vi "Init.vi"(8 "error in (no error)":errorcluster, 11 "reference in":refnum<class "Test_Flux_Capacitor.lvclass">) -> (0 "error out":errorcluster, 3 "reference out":refnum<class "Test_Flux_Capacitor.lvclass">)   [LabVIEW 2022 SP3, in "Test_Flux_Capacitor.lvlib" / "Test_Flux_Capacitor.lvclass"]
uses:
  Test_Flux_Capacitor.lvclass
  Components/Test_Base.lvlibp/Test_Base.lvclass
  Components/ViPER.lvlibp/ViPER.lvclass
  C:/Projects/Medulla/ViPER/Examples/Flux_Capacitor_Tester/Components/ViPER.lvlibp/ViPER.lvclass
  Components/Flux_Capacitor.lvlibp/Flux_Capacitor.lvclass
  Components/SwitchBase.lvlibp/SwitchBase.lvclass
  Components/PSU_Base.lvlibp/PSU_Base.lvclass
  Components/LCR_BK891.lvlibp/LCR_BK891.lvclass
  Components/DMM_Keysight_34980A.lvlibp/DMM_Keysight_34980A.lvclass
  Components/JTAG_Base.lvlibp/JTAG_Base.lvclass
  Components/Frequency_Counter_Base.lvlibp/Frequency_Counter_Base.lvclass
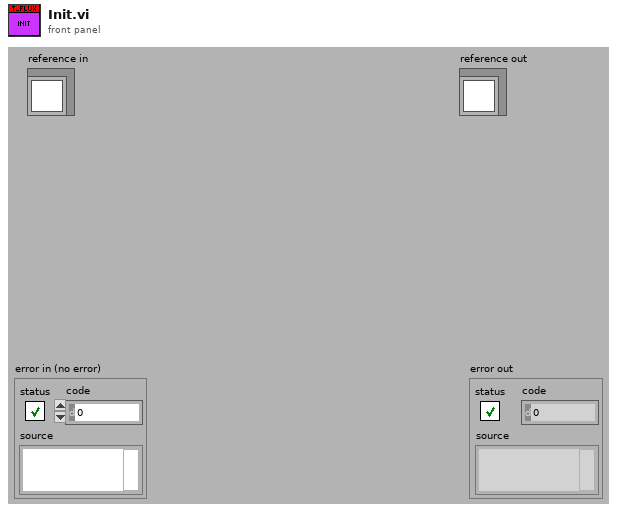
[diagram p1: front panel]
types:
  T1 = typedef "Test_Flux_Capacitor.lvlib/Test_Flux_Capacitor.lvclass/ObjectAttributes.ctl" = cluster{"Config":T2, "DMM":refnum<class "DMM_Keysight_34980A.lvclass">, "LCR":refnum<class "LCR_BK891.lvclass">, "PSU":refnum<class "PSU_Base.lvclass">, "Switch_Manager":refnum<class "SwitchBase.lvclass">, "FRAM":string, "Flux_Capacitor":refnum<class "Flux_Capacitor.lvclass">, "Frequency_Counter":refnum<class "Frequency_Counter_Base.lvclass">, "JTAG":refnum<class "JTAG_Base.lvclass">}
  T2 = typedef "Test_Flux_Capacitor.lvlib/Test_Flux_Capacitor.lvclass/Config.ctl" = cluster{"default":string}
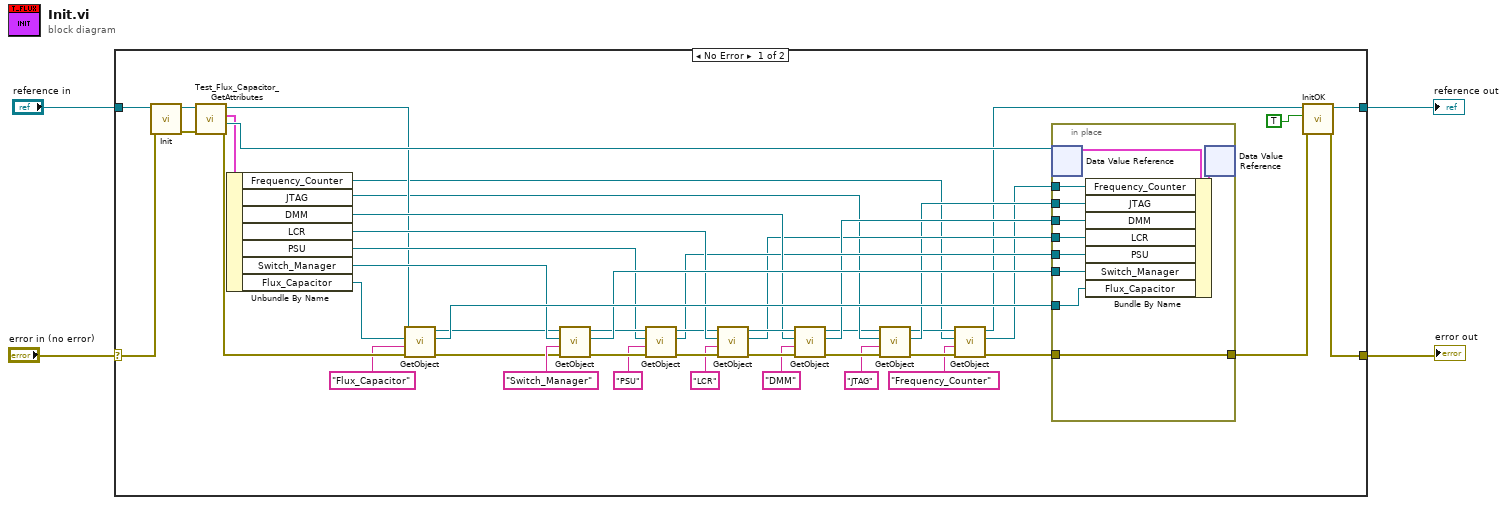
[diagram p0: block diagram]
diagram:
  n1 = case shown="No Error" "error in (no error)" {
    selector: "error in (no error)" -> [w50 w63]
    tunnel: [w43 w63] -> w3
    tunnel: [w46 w62] -> w1
    tunnel: "reference in" -> [w51 w62]
    frame No Error {
      n2 = call-parent "Init.vi"("error in (no error)"=w50, "reference in"=w51) -> ("error out"=w48:errorcluster, "reference out"=w49:refnum<class "Test_Flux_Capacitor.lvclass">)  [unwired: 8 in]
      n3 = call "Test_Flux_Capacitor_GetAttributes.vi"("error in (no error)"=w48, "reference in"=w49) -> ("error out"=w42:errorcluster, "DataRef"=w47:refnum<data-value>, "Data"=w41:T1, "reference out"=w19:refnum<class "Test_Flux_Capacitor.lvclass">)  [unwired: 6 in]
      n4 = Unbundle By Name(w41) -> ("Frequency_Counter"=w8:refnum<class "Frequency_Counter_Base.lvclass">, "JTAG"=w15:refnum<class "JTAG_Base.lvclass">, "DMM"=w24:refnum<class "DMM_Keysight_34980A.lvclass">, "LCR"=w29:refnum<class "LCR_BK891.lvclass">, "PSU"=w32:refnum<class "PSU_Base.lvclass">, "Switch_Manager"=w37:refnum<class "SwitchBase.lvclass">, "Flux_Capacitor"=w40:refnum<class "Flux_Capacitor.lvclass">)
      n5 = call "GetObject.vi"("error in (no error)"=w42, "Object Name"="Flux_Capacitor", "Class type"=w40, "reference in"=w19) -> ("error out"=w18:errorcluster, "Object out"=w38:refnum<class "Flux_Capacitor.lvclass">, "reference out"=w17:refnum<class "Test_Flux_Capacitor.lvclass">)  [unwired: 5 in]
      n6 = call "GetObject.vi"("error in (no error)"=w18, "Object Name"="Switch_Manager", "Class type"=w37, "reference in"=w17) -> ("error out"=w34:errorcluster, "Object out"=w35:refnum<class "SwitchBase.lvclass">, "reference out"=w33:refnum<class "Test_Flux_Capacitor.lvclass">)  [unwired: 5 in]
      n7 = call "GetObject.vi"("error in (no error)"=w34, "Object Name"="PSU", "Class type"=w32, "reference in"=w33) -> ("error out"=w30:errorcluster, "Object out"=w22:refnum<class "PSU_Base.lvclass">, "reference out"=w28:refnum<class "Test_Flux_Capacitor.lvclass">)  [unwired: 5 in]
      n8 = call "GetObject.vi"("error in (no error)"=w30, "Object Name"="LCR", "Class type"=w29, "reference in"=w28) -> ("error out"=w26:errorcluster, "Object out"=w20:refnum<class "LCR_BK891.lvclass">, "reference out"=w25:refnum<class "Test_Flux_Capacitor.lvclass">)  [unwired: 5 in]
      n9 = call "GetObject.vi"("error in (no error)"=w26, "Object Name"="DMM", "Class type"=w24, "reference in"=w25) -> ("error out"=w16:errorcluster, "Object out"=w21:refnum<class "DMM_Keysight_34980A.lvclass">, "reference out"=w14:refnum<class "Test_Flux_Capacitor.lvclass">)  [unwired: 5 in]
      n10 = call "GetObject.vi"("error in (no error)"=w16, "Object Name"="JTAG", "Class type"=w15, "reference in"=w14) -> ("error out"=w11:errorcluster, "Object out"=w13:refnum<class "JTAG_Base.lvclass">, "reference out"=w9:refnum<class "Test_Flux_Capacitor.lvclass">)  [unwired: 5 in]
      n11 = call "GetObject.vi"("error in (no error)"=w11, "Object Name"="Frequency_Counter", "Class type"=w8, "reference in"=w9) -> ("error out"=w10:errorcluster, "Object out"=w7:refnum<class "Frequency_Counter_Base.lvclass">, "reference out"=w6:refnum<class "Test_Flux_Capacitor.lvclass">)  [unwired: 5 in]
      n12 = in-place {
        in-place-border: w10 -> [w61]
        in-place-border: [w61] -> w44
        in-place-border: w38 -> [w58]
        in-place-border: w35 -> [w57]
        in-place-border: w22 -> [w56]
        in-place-border: w21 -> [w55]
        in-place-border: w20 -> [w54]
        in-place-border: w13 -> [w53]
        in-place-border: w7 -> [w52]
        n13 = in-place-dvr #1(w47) -> (w60:T1)  [unwired: 1 out]
        n14 = Bundle By Name(cluster=w60, "Frequency_Counter"=w52, "JTAG"=w53, "DMM"=w55, "LCR"=w54, "PSU"=w56, "Switch_Manager"=w57, "Flux_Capacitor"=w58) -> (w59:T1)
        n15 = in-place-dvr #1(w59) -> ()  [unwired: 2 out]
      }
      n16 = call "InitOK.vi"("error in (no error)"=w44, "Init OK?"=TRUE, "reference in"=w6) -> ("error out"=w43:errorcluster, "reference out"=w46:refnum<class "Test_Flux_Capacitor.lvclass">)  [unwired: 7 in]
    }
    frame Error {
    }
  }
  "error out" <- w3
  "reference out" <- w1
